vi "Utility Format User Compensation.vi"(8 "error in (no error)":errorcluster, 11 "Compensation (%)":dbl) -> (0 "error out":errorcluster, 3 "Formatted Compensation":string)   [LabVIEW 2020, in "ChromTech MX-Class Drivers.lvlib"]
doc: "Formats the command to set the User Compensation, given a desired compensation number. This number must be between 85.0 and 115.0, or the function will default to a compensation value of 100.0."
uses:
  <instrlib>/RxnRover/ChromtechNextGenDriver/ChromTech MX-Class Drivers.lvlib
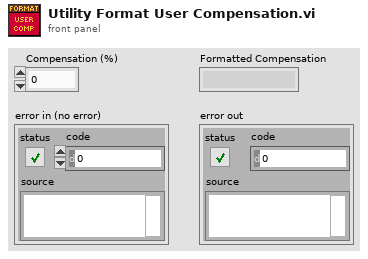
[diagram p1: front panel]
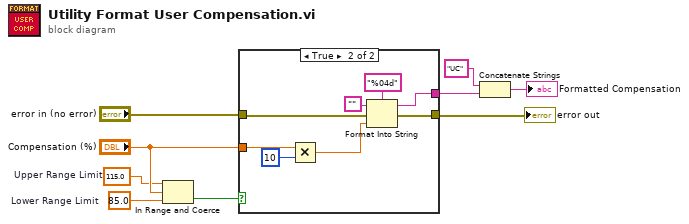
[diagram p0: block diagram]
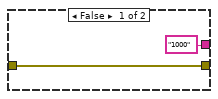
[diagram p2: hidden frame]
diagram:
  w3 = 115.0  # Upper Range Limit
  w2 = 85.0  # Lower Range Limit
  n1 = In Range and Coerce(upper limit=w3, x="Compensation (%)", lower limit=w2) -> (In Range?=w1:bool)  [unwired: 1 out]
  n2 = case shown="True" w1 {
    tunnel: "error in (no error)" -> [w11 w18]
    tunnel: "Compensation (%)" -> [_ w14]
    tunnel: [w11 w17] -> w9
    tunnel: ["1000" w16] -> w5
    frame False {
    }
    frame True {
      n3 = Multiply(x=w14, y=10) -> (x*y=w13:dbl)
      n4 = Format Into String(format string="%04d", initial string="", error in=w18, w13) -> (resulting string=w16:string, error out=w17:errorcluster)
    }
  }
  "error out" <- w9
  n5 = Concatenate Strings("UC", w5) -> (→"Formatted Compensation":string)
